vi "get default exposure time.vi"(8 "error in (no error)":errorcluster, 11 "Thorcam in":refnum<class "Thorcam.lvclass">) -> (0 "error out":errorcluster, 1 "exposure time":dbl[unit], 3 "Thorcam out":refnum<class "Thorcam.lvclass">)   [LabVIEW 2012, in "Thorcam.lvclass"]
uses:
  Thorcam.lvclass
  Thorcam.lvclass/Thorcam.ctl
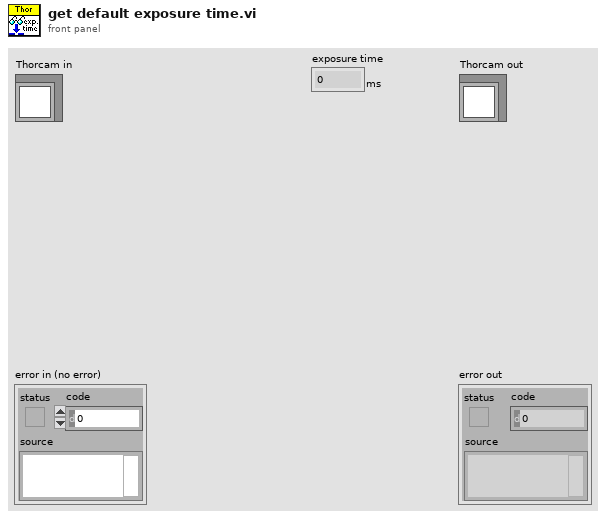
[diagram p1: front panel]
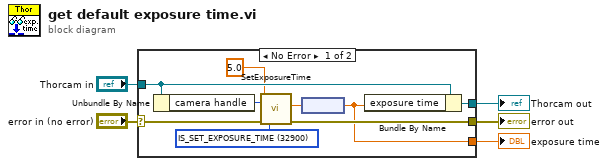
[diagram p0: block diagram]
diagram:
  n1 = case shown="No Error" "error in (no error)" {
    selector: "error in (no error)" -> [w13 w16]
    tunnel: [w12 w16] -> w4
    tunnel: [w9 w15] -> w2
    tunnel: "Thorcam in" -> [w10 w15]
    tunnel: [w7 _] -> w1
    frame No Error {
      w11 = u16 32900 items=["IS_SET_EXPOSURE_TIME"=32900, "IS_GET_EXPOSURE_TIME"=32768, "IS_GET_DEFAULT_EXPOSURE"=32769] ("Mode")
      n2 = Unbundle By Name(w10) -> ("camera handle"=w14:u32)
      n3 = call <instrlib>:"SetExposureTime.vi"("error in"=w13, "Mode"=w11, "Exposure Time"=5.0, "Camera Handle In"=w14) -> ("error out"=w12:errorcluster, "new exposure time"=w8:dbl)  [unwired: 5 in, 1 out]
      n4 = node(w8) -> (w7:dbl[unit])
      n5 = Bundle By Name(cluster=w10, "exposure time"=w7) -> (w9:refnum<class "Thorcam.lvclass">)
    }
    frame Error {
    }
  }
  "error out" <- w4
  "Thorcam out" <- w2
  "exposure time" <- w1
